vi "ChangeButtonsStateExcept.vi"(9 "Disabled":T1(ring)=enum."Disabled and Grayed Out", 10 "Exceptions":refnum<vi>[](array[refnum]), 11 "VI in":refnum<vi>) -> ()   [LabVIEW 2023, in "InterferometrUI.lvlib" / "InterferometerUI.lvclass"]
uses:
  InterferometerUI.lvclass
  InterferometerUI.lvclass/InterferometerUI.ctl
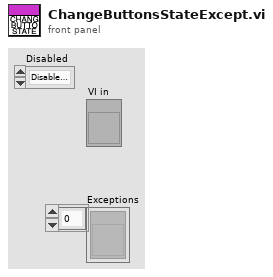
[diagram p1: front panel]
types:
  T1 = enum8{"Enabled", "Disabled", "Disabled and Grayed Out"}
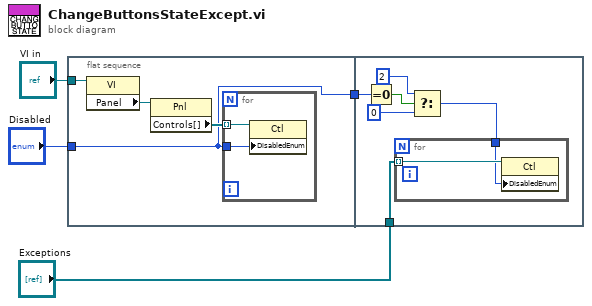
[diagram p0: block diagram]
diagram:
  n1 = flat-sequence {
    tunnel: "VI in" -> [w6]
    tunnel: "Disabled" -> [w5]
    tunnel: [w5] -> w1
    tunnel: "Exceptions" -> [w16]
    tunnel: w1 -> [w14]
    frame #0 {
      n2 = property on="Property Node" class="VI"(reference=w6) -> ("Panel"=w8:refnum<vi>)  [unwired: 1 in, 2 out]
      n3 = property on="Property Node" class="Pnl"(reference=w8) -> ("Controls[]"=w7:refnum<vi>[])  [unwired: 1 in, 2 out]
      n4 = for {
        tunnel: w7 -> [w10] mode=indexing
        tunnel: w5 -> [w9]
        n5 = property on="Property Node" class="Ctl"(reference=w10, "DisabledEnum"=w9) -> ()  [unwired: 1 in, 2 out]
      }
    }
    frame #1 {
      n6 = Equal To 0?(x=w14) -> (x = 0?=w15:bool)
      n7 = Select(t=2, s=w15, f=0) -> (s? t:f=w11:i32)
      n8 = for {
        tunnel: w16 -> [w18] mode=indexing
        tunnel: w11 -> [w17]
        n9 = property class="Ctl"(reference=w18, "DisabledEnum"=w17) -> ()  [unwired: 1 in, 2 out]
      }
    }
  }
